vi "add dataset.vi"(9 "fields":string[](array[string]), 10 "name":string, 11 "folder":string[](array[string])) -> (0 "error out":errorcluster, 3 "path":string[](array[string]))   [LabVIEW 2014]
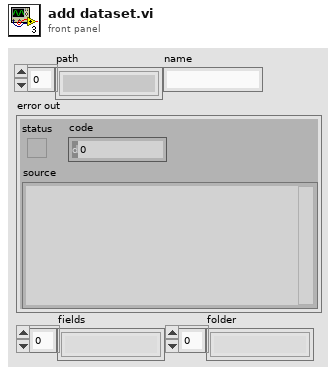
[diagram p1: front panel]
types:
  T1 = cluster{"fields":string[], "folder":string[], "name":string}
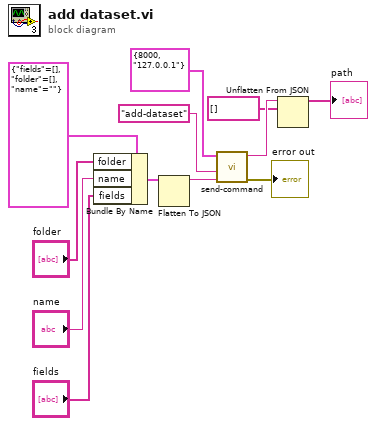
[diagram p0: block diagram]
diagram:
  n1 = Bundle By Name(cluster=T1 {"fields"=[], "folder"=[], "name"=""}, "folder"="folder", "name"="name", "fields"="fields") -> (w1:T1)
  n2 = Flatten To JSON(anything=w1) -> (JSON string=w6:string)  [unwired: 2 in, 1 out]
  n3 = call "send-command.vi"("parameters"=w6, "command"="add-dataset", "target"=cluster{"port":i32, "host":string} {"port"=8000, "host"="127.0.0.1"}) -> ("error out"=→"error out":errorcluster, "output"=w10:string)  [unwired: 7 in]
  n4 = Unflatten From JSON(JSON string=w10, type and defaults=string[] []) -> (value=→"path":string[])  [unwired: 5 in, 1 out]
